vi "Convert To Driver DataType.vi"(8 "error in":errorcluster, 10 "In":dbl) -> (0 "error out":errorcluster, 2 "Out":i32)   [LabVIEW 2026, in "Runtime Configuration Support Example Engine.lvlib"]
uses:
  Runtime Configuration Support Example Engine.lvlib
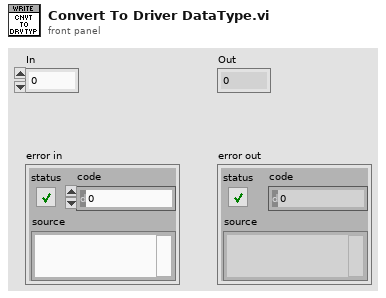
[diagram p1: front panel]
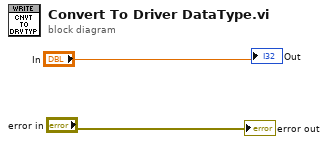
[diagram p0: block diagram]
diagram:
  "Out" <- "In"
  "error out" <- "error in"
